vi "Measurement UI.vi"() -> ()   [LabVIEW 2021, in "Load Transient Response with Pin Map UI.lvlib"]
uses:
  Load Transient Response with Pin Map UI.lvlib
  common/builds/PMIC Common.lvlibp/UI/controls/Open Dialog.ctl
  <instrlib>/niScope/Controls/niScope vertical coupling.ctl
  common/builds/PMIC Common.lvlibp/UI/controls/UI Scope Parameters.ctl
  646e44c3-9b14-4556-aaa1-803f5bf26e68.vi
  common/builds/PMIC Common.lvlibp
panel:
  in  "MeasGraphs":T1(tab)
  out "MeasTable":string[][](table)
  out "LoadCurrentV/STimeGraph":waveform(dbl)(graph) caption="Load Transient"
  out "OutputVoltageV/STimeGraph":waveform(dbl)(graph) caption="Load Transient"
  in  "Load Current v/s Time":string="LOAD CURRENT vs TIME"
  in  "Output Voltage v/s Time":string="LOAD VOLTAGE vs TIME"
  out "ScopeGraph":T2(graph)
  out "waveform pins":string[](array[string])
  in  "enforce realtime":bool[](array[boolean])
  in  "reference position":dbl[](array[numeric]) caption="MIN SAMPLE RATE"
  in  "channel enabled":bool[](array[boolean])
  out "waveform length array":i32[](array[numeric])
  out "waveform dt array":dbl[](array[numeric])
  out "concatenated waveform Y":dbl[](array[numeric])
  out "waveform t0 array":dbl[](array[numeric])
  out "waveform sites":i32[](array[numeric])
  in  "vertical range":dbl[](array[numeric]) caption="VERTICAL RANGE"
  in  "vertical offset":dbl[](array[numeric]) caption="VERTICAL OFFSET"
  in  "probe attenuation":dbl[](array[numeric]) caption="PROBE ATTENUATION"
  in  "vertical coupling":T3[](array[typedef]) caption="VERTICAL COUPLING" items=["AC", "DC", "Ground"]
  in  "input impedance":u32[](array[ring]) caption="INPUT IMPEDANCE" items=["1 mega ohm"=0, "50 ohms"=2]
  in  "max input frequency":dbl[](array[numeric]) caption="MAX INPUT FREQUENCY"
  in  "min sample rate":dbl[](array[numeric]) caption="MIN SAMPLE RATE"
  in  "min record length":i32[](array[numeric]) caption="MIN RECORD LENGTH"
  in  "Pin Names for Scope":string[](array[string]) caption="PIN NAMES"
  out "Overshoot load voltage":dbl
  out "Undershoot load voltage":dbl
  out "dt":dbl
  out "Load voltages":dbl[](array[numeric])
  out "Load currents":dbl[](array[numeric])
  in  "Source transient response":i32(ring)=1042 items=["Slow"=1041, "Normal"=1038, "Fast"=1039, "Custom"=1042]
  in  "Load transient response":i32(ring)=3 items=["Slow"=1041, "Normal"=1038, "Fast"=1039, "Custom"=1042]
  in  "Open Dialog":T4
  in  "Scope configuration":string="Scope configuration"
  in  "Load pin name":string caption="LOAD PIN NAME"
  in  "Source pin name":string caption="SOURCE PIN NAME"
  in  "Load sense":i32(ring)=1009 caption="SENSE" items=["Local"=1008, "Remote"=1009]
  in  "Source sense":i32(ring)=1009 caption="SENSE" items=["Local"=1008, "Remote"=1009]
  in  "Load current delay t2":dbl=0.001 caption="DELAY T2" format="%#_6ps"
  in  "Load current delay t1":dbl=0.001 caption="DELAY T1" format="%#_6ps"
  in  "Load current pulse duration":dbl=0.001 caption="PULSE DURATION" format="%#_6ps"
  in  "Load current level range":dbl=40.0 caption="CURRENT LEVEL RANGE" format="%#_6pA"
  in  "Load current rising slew rate":dbl=24.0 caption="CURRENT RISING SLEW RATE" format="%#_6pA/us"
  in  "Load current falling slew rate":dbl=24.0 caption="CURRENT FALLING SLEW RATE" format="%#_6pA/us"
  in  "Load configuration":string="Load configuration"
  in  "Source configuration":string="Source configuration"
  in  "Source voltage level":dbl=12.0 caption="VOLTAGE LEVEL" format="%#_6pV"
  in  "Source current limit":dbl=25.0 caption="CURRENT LIMIT" format="%#_6pA"
  in  "Source voltage pole-zero ratio":dbl=2.0 caption="POLE-ZERO RATIO"
  in  "Source voltage gain bandwidth":dbl=2000.0 caption="GAIN BANDWIDTH" format="%#_6pHz"
  in  "Source voltage compensation frequency":dbl=3530.0 caption="COMP. FREQUENCY" format="%#_6pHz"
  in  "Source fast":bool
  in  "Source normal":bool
  in  "Source slow":bool
  in  "Source SourceAdapt":string="Voltage SourceAdapt Parameters"
  in  "Load voltage limit range":dbl=6.0 caption="VOLTAGE LIMIT RANGE" format="%#_6pV"
  in  "Load current set point 1":dbl=4.0 caption="CURRENT SET POINT 1" format="%#_6pA"
  in  "Load current pole-zero ratio":dbl=0.3 caption="POLE-ZERO RATIO"
  in  "Load current gain bandwidth":dbl=14000.0 caption="GAIN BANDWIDTH" format="%#_6pHz"
  in  "Load current compensation frequency":dbl=180000.0 caption="COMP. FREQUENCY" format="%#_6pHz"
  in  "Load sample rate":dbl=1800000.0 caption="SAMPLE RATE" format="%#_6pS/s"
  in  "Load current set point 2":dbl=14.0 caption="CURRENT SET POINT 2" format="%#_6pA"
  in  "Load fast":bool
  in  "Load normal":bool
  in  "Load slow":bool
  in  "Load SourceAdapt":string="Current SourceAdapt Parameters"
  out "Status":string
  in  "DUT setup time":dbl=1.0 caption="DUT SETUP TIME" format="%#_6ps"
  in  "Measurement settings":string="Measurement settings"
  in  "Nominal output voltage":dbl=3.3 caption="NOMINAL OUTPUT VOLTAGE" format="%#_6pV"
  in  "Mode of operation":T5(ring)=enum."Perform measurement" caption="MODE OF OPERATION"
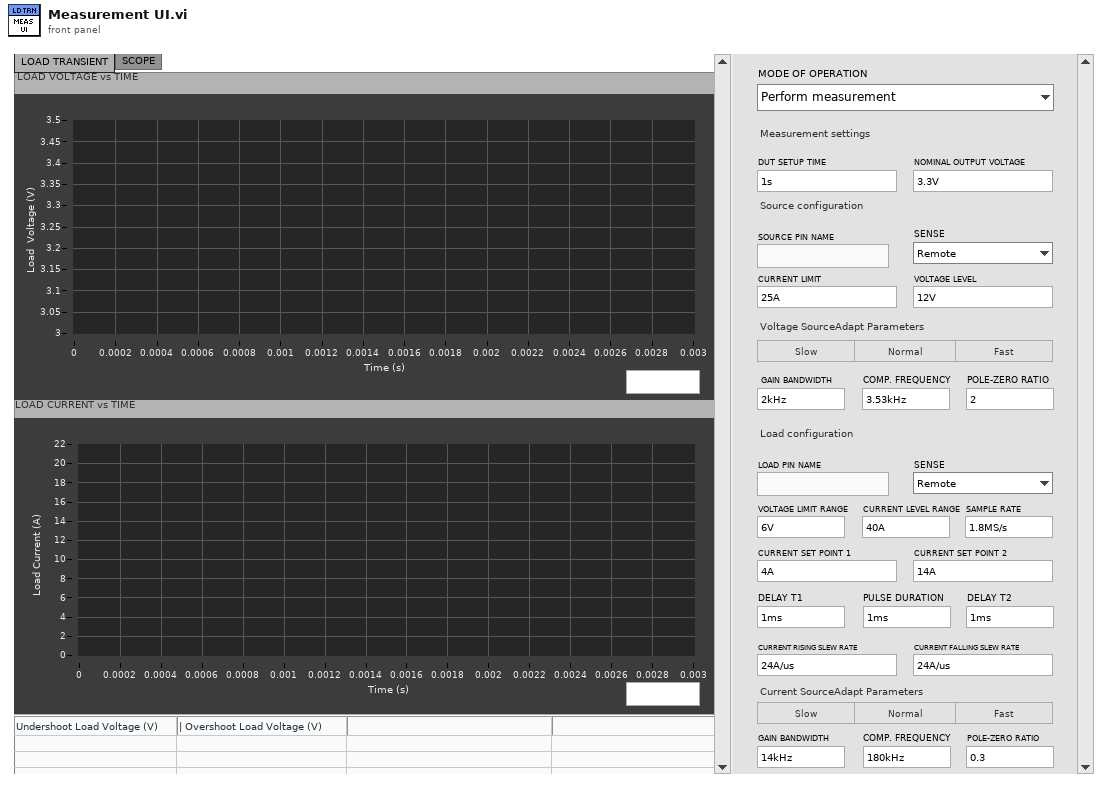
[diagram p1: front panel]
types:
  T1 = enum32{"LOAD TRANSIENT", "SCOPE", "Hidden Controls"}
  T2 = cluster{"Load currents":dbl[], "Efficiency":dbl[]}[]
  T3 = typedef "niScope vertical coupling.ctl" = i32
  T4 = typedef "PMIC Common.lvlibp/Open Dialog.ctl" = bool
  T5 = enum32{"Power on the DUT", "Perform measurement", "Power off the DUT"}
  T6 = typedef "PMIC Common.lvlibp/UI Scope Parameters.ctl" = cluster{"Pin name":string, "Vertical range":dbl, "Vertical offset":dbl, "Probe attenuation":dbl, "Vertical coupling":i32, "Channel enabled":bool, "Input impedance":u32, "Max input frequency":dbl, "Min sample rate":dbl, "Reference position":dbl, "Min record length":i32, "Enforce realtime":bool}
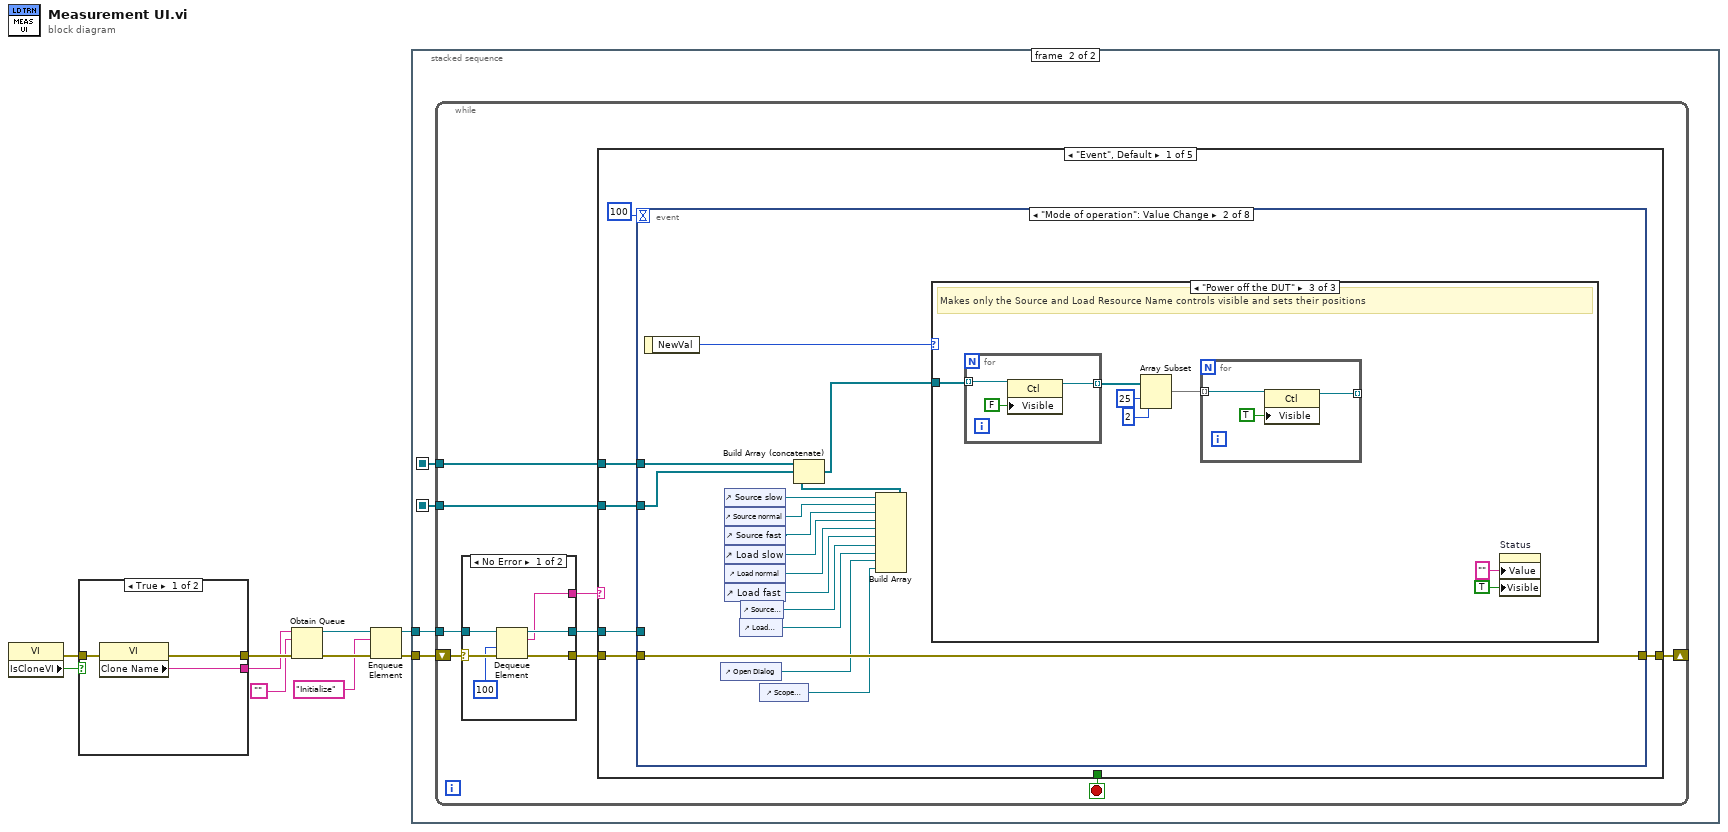
[diagram p0: block diagram]
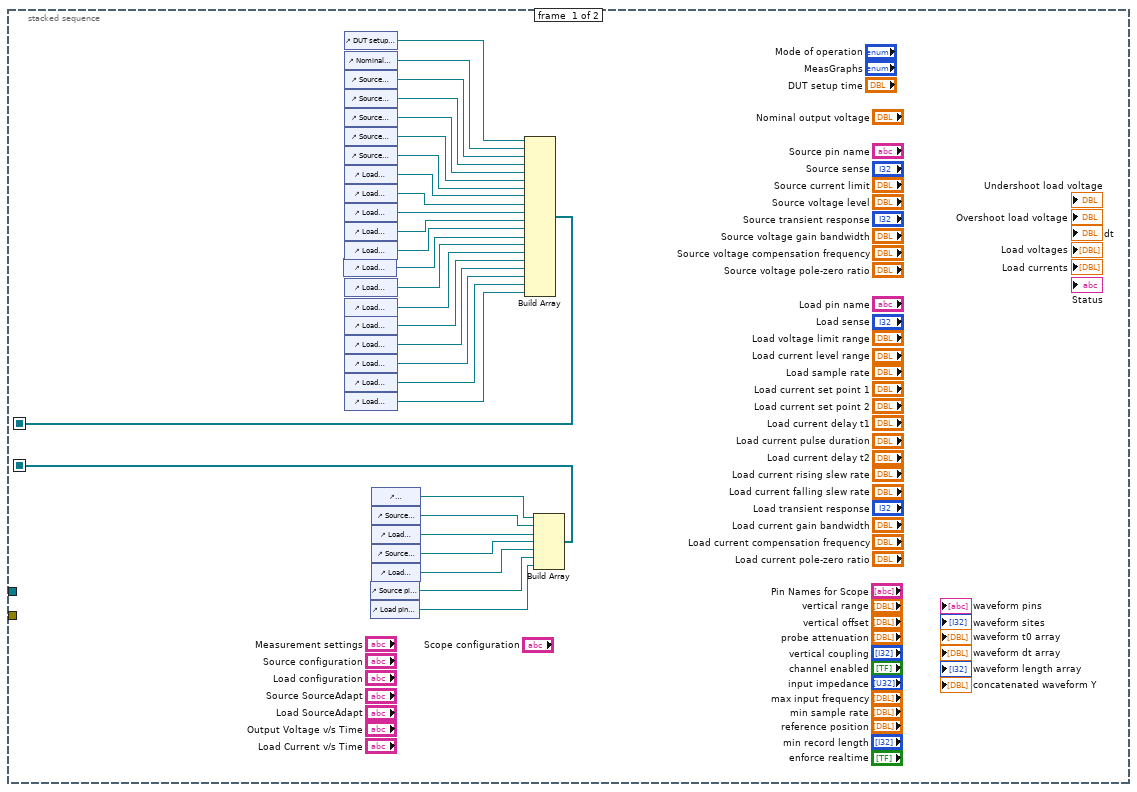
[diagram p2: hidden frame]
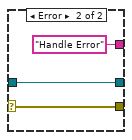
[diagram p3: hidden frame]
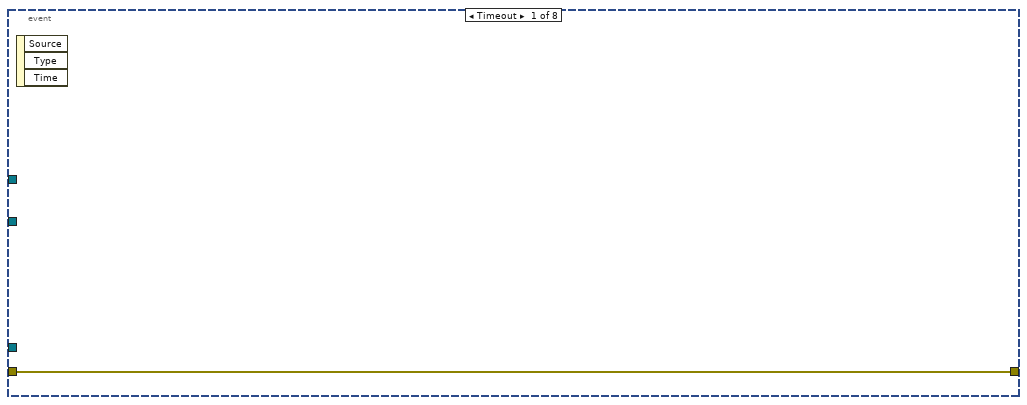
[diagram p4: hidden frame]
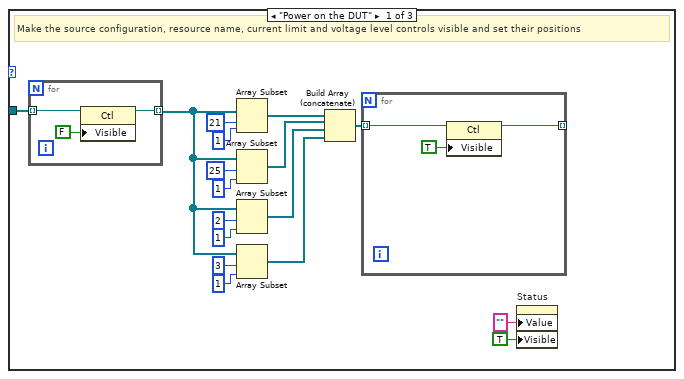
[diagram p5: hidden frame]
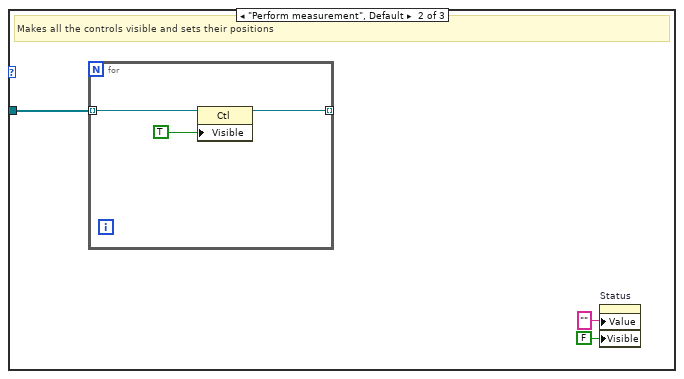
[diagram p6: hidden frame]
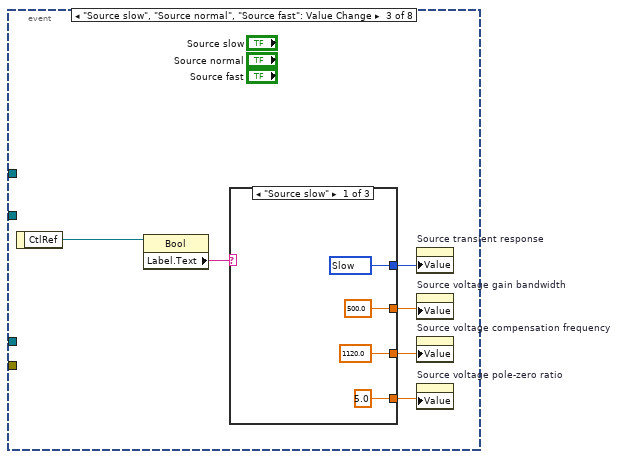
[diagram p7: hidden frame]
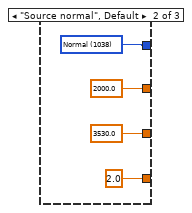
[diagram p8: hidden frame]
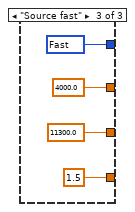
[diagram p9: hidden frame]
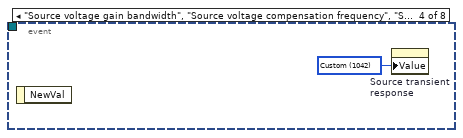
[diagram p10: hidden frame]
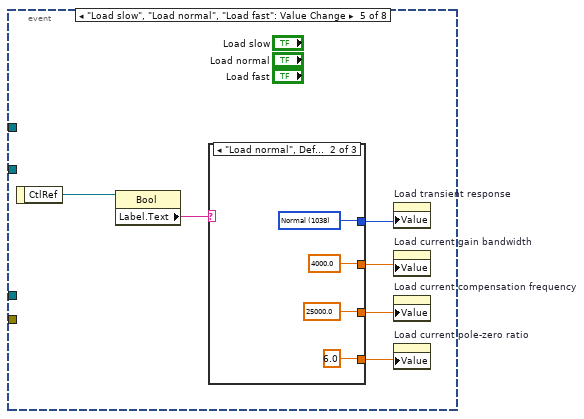
[diagram p11: hidden frame]
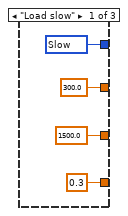
[diagram p12: hidden frame]
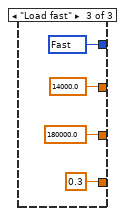
[diagram p13: hidden frame]
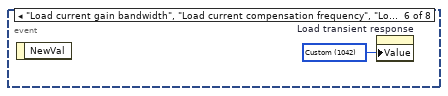
[diagram p14: hidden frame]
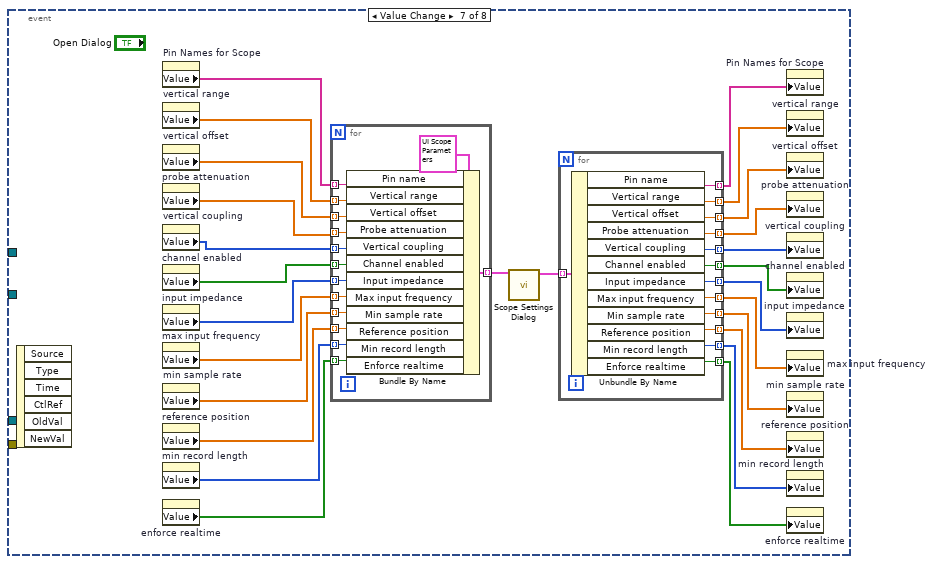
[diagram p15: hidden frame]
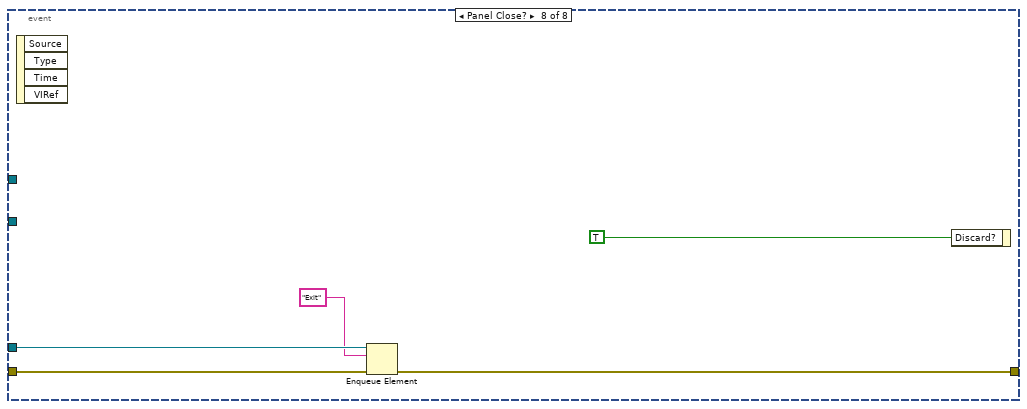
[diagram p16: hidden frame]
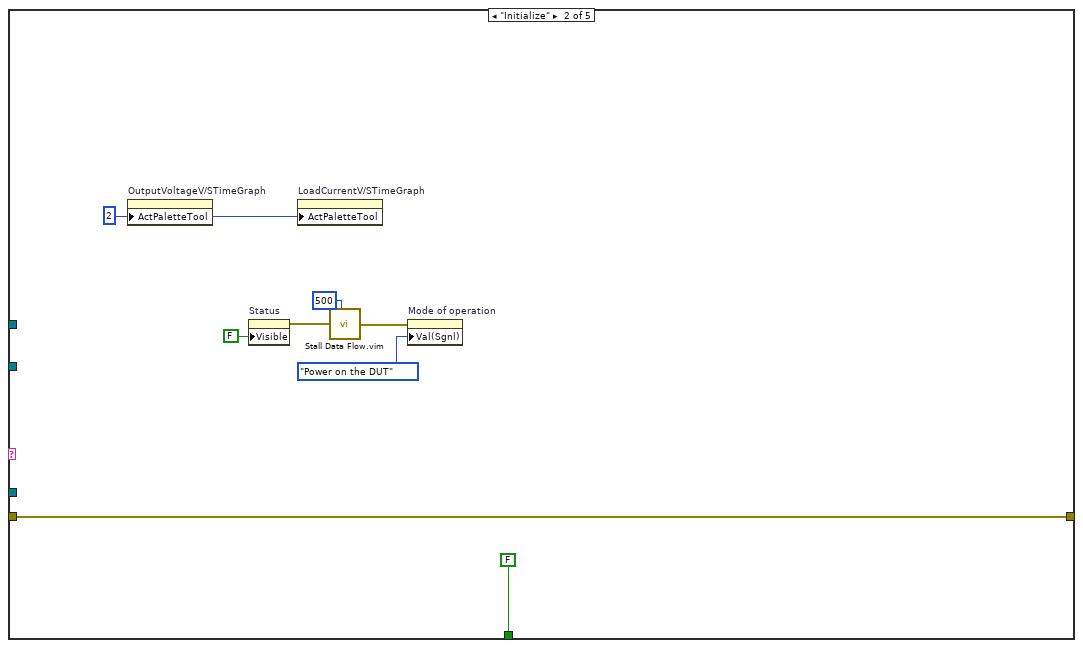
[diagram p17: hidden frame]
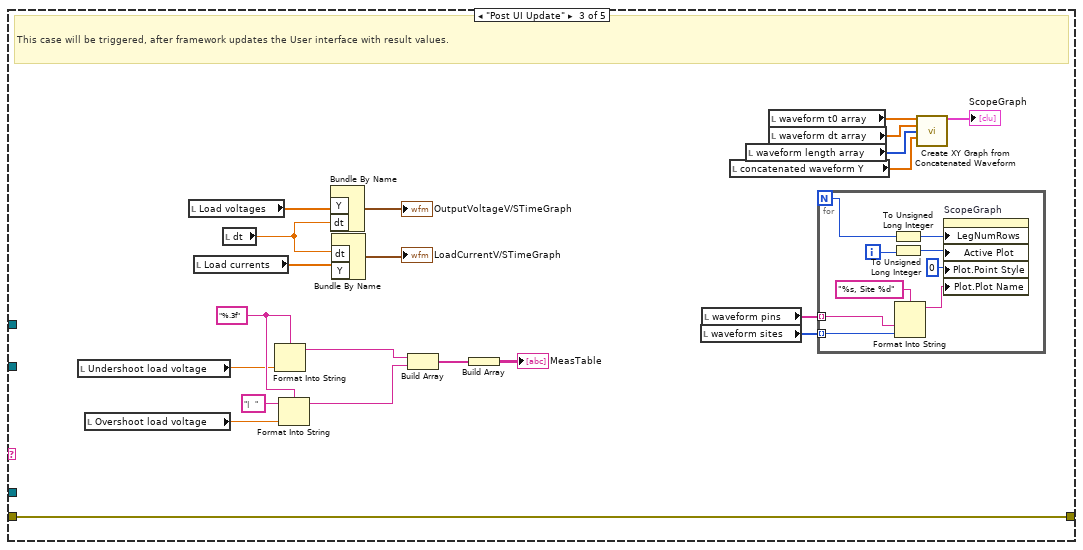
[diagram p18: hidden frame]
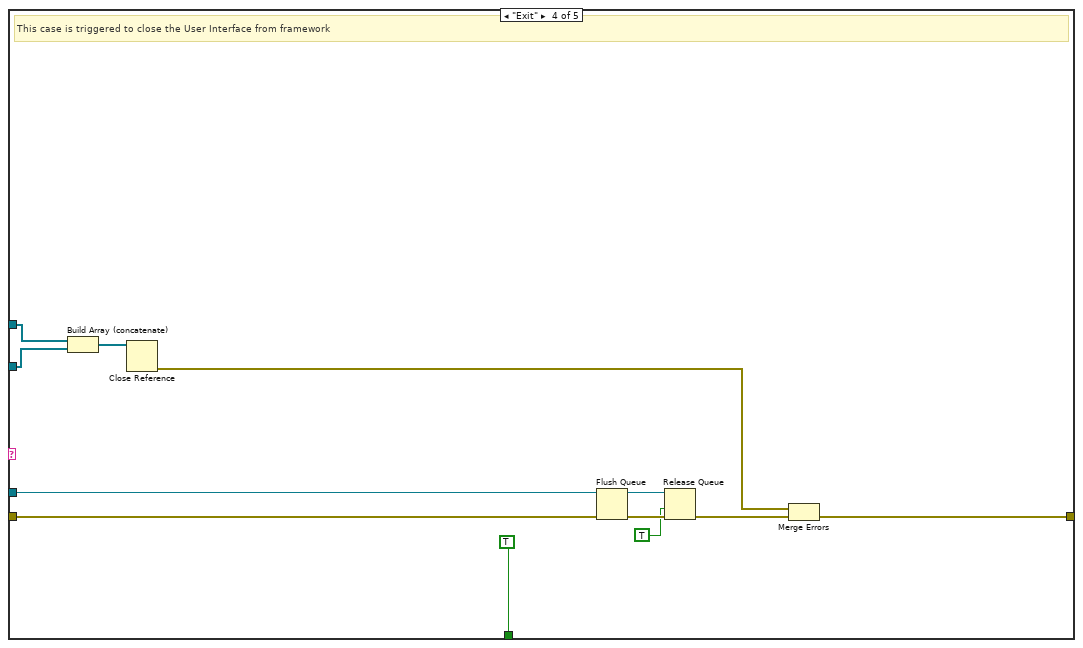
[diagram p19: hidden frame]
diagram:
  n1 = property class="VI"() -> (error out=w1:errorcluster, "IsCloneVI"=w2:bool)  [unwired: 2 in, 1 out]
  n2 = case shown="True" w2 {
    tunnel: [w13 w16] -> w10
    tunnel: [w12 w15] -> w9
    tunnel: w1 -> [w11 w14]
    frame True {
      n3 = property class="VI"(error in=w11) -> (error out=w13:errorcluster, "Clone Name"=w12:string)  [unwired: 1 in, 1 out]
    }
    frame False {
      n4 = property class="VI"(error in=w14) -> (error out=w16:errorcluster, "Name"=w15:string)  [unwired: 1 in, 1 out]
    }
  }
  n5 = Obtain Queue(name (unnamed)=w9, element data type="", error in (no error)=w10) -> (queue out=w6:refnum<queue>, error out=w8:errorcluster)  [unwired: 2 in, 1 out]
  n6 = Enqueue Element(queue=w6, element="Initialize", error in (no error)=w8) -> (queue out=w5:refnum<queue>, error out=w7:errorcluster)  [unwired: 1 in, 1 out]
  n7 = stacked-sequence {
    seq-local: [w31 _] -> [_ w47]
    seq-local: [w32 _] -> [_ w46]
    tunnel: w7 -> [_ w49]
    tunnel: w5 -> [_ w48]
    frame #0 {
      n8 = control-ref of="Load current delay t1"() -> (w21:refnum<vi>)
      n9 = control-ref of="DUT setup time"() -> (w24:refnum<vi>)
      n10 = control-ref of="Nominal output voltage"() -> (w45:refnum<vi>)
      n11 = control-ref of="Source current limit"() -> (w44:refnum<vi>)
      n12 = control-ref of="Source voltage level"() -> (w43:refnum<vi>)
      n13 = control-ref of="Source voltage gain bandwidth"() -> (w42:refnum<vi>)
      n14 = control-ref of="Source voltage compensation frequency"() -> (w41:refnum<vi>)
      n15 = control-ref of="Source voltage pole-zero ratio"() -> (w40:refnum<vi>)
      n16 = control-ref of="Load voltage limit range"() -> (w39:refnum<vi>)
      n17 = control-ref of="Load current level range"() -> (w26:refnum<vi>)
      n18 = control-ref of="Load sample rate"() -> (w38:refnum<vi>)
      n19 = control-ref of="Load current set point 1"() -> (w37:refnum<vi>)
      n20 = control-ref of="Load current set point 2"() -> (w36:refnum<vi>)
      n21 = control-ref of="Load current pulse duration"() -> (w20:refnum<vi>)
      n22 = control-ref of="Load current delay t2"() -> (w19:refnum<vi>)
      n23 = control-ref of="Load current rising slew rate"() -> (w22:refnum<vi>)
      n24 = control-ref of="Load current falling slew rate"() -> (w23:refnum<vi>)
      n25 = control-ref of="Load current gain bandwidth"() -> (w25:refnum<vi>)
      n26 = control-ref of="Load current compensation frequency"() -> (w35:refnum<vi>)
      n27 = control-ref of="Load current pole-zero ratio"() -> (w33:refnum<vi>)
      n28 = control-ref of="Source pin name"() -> (w18:refnum<vi>)
      n29 = control-ref of="Load pin name"() -> (w17:refnum<vi>)
      n30 = control-ref of="Measurement settings"() -> (w34:refnum<vi>)
      n31 = control-ref of="Source configuration"() -> (w30:refnum<vi>)
      n32 = control-ref of="Load configuration"() -> (w29:refnum<vi>)
      n33 = control-ref of="Source SourceAdapt"() -> (w28:refnum<vi>)
      n34 = control-ref of="Load SourceAdapt"() -> (w27:refnum<vi>)
      n35 = Build Array(w24, w45, w44, w43, w42, w41, w40, w39, w26, w38, w37, w36, w21, w20, w19, w22, w23, w25, w35, w33) -> (w31:refnum<vi>[])
      n36 = Build Array(w34, w30, w29, w28, w27, w18, w17) -> (w32:refnum<vi>[])
    }
    frame #1 {
      n37 = while {
        shift-right: [w53] -> _
        shift-left: w49 -> [w58]
        tunnel: w48 -> [w56]
        tunnel: w47 -> [w51]
        tunnel: w46 -> [w50]
        stop <- w52 stop-if-true
        n38 = case shown="No Error" w58 {
          selector: w58 -> [w64 w67]
          tunnel: [w63 w67] -> w57
          tunnel: w56 -> [w62 w66]
          tunnel: [w61 w66] -> w55
          tunnel: [w60 "Handle Error"] -> w54
          frame No Error {
            n39 = Dequeue Element(queue=w62, timeout in ms (-1)=100, error in (no error)=w64) -> (queue out=w61:refnum<queue>, element=w60:string, error out=w63:errorcluster)  [unwired: 1 out]
          }
          frame Error {
          }
        }
        n40 = case shown="\"Event\", Default" w54 {
          tunnel: w57 -> [w72 w236 w257 w278 w279]
          tunnel: w55 -> [w70 _ _ w276 _]
          tunnel: [w73 w236 w257 w267 w279] -> w53
          tunnel: [_ FALSE _ TRUE _] -> w52
          tunnel: w51 -> [w69 _ _ w272 _]
          tunnel: w50 -> [w68 _ _ w271 _]
          frame "Event", Default {
            n41 = event shown="[1] \"Mode of operation\": Value Change" {
              selector: _ -> [_ _ _ _ _ _ _ _]
              dyn-events: _ -> [_ _ _ _ _ _ _ _]
              timeout: 100 -> [_ _ _ _ _ _ _ _]
              tunnel: [w74 w86 _ _ _ _ _ w226] -> w73
              tunnel: w72 -> [w74 w86 _ _ _ _ _ w227]
              tunnel: w70 -> [_ _ _ _ _ _ _ w225]
              tunnel: w69 -> [_ w88 _ _ _ _ _ _]
              tunnel: w68 -> [_ w87 _ _ _ _ _ _]
              event Timeout {
                n42 = event-data() -> ()  [unwired: 1 in, 3 out]
              }
              event "Mode of operation": Value Change {
                n43 = event-data() -> ("NewVal"=w90:T5)  [unwired: 1 in]
                n44 = control-ref of="Open Dialog"() -> (w76:refnum<vi>)
                n45 = control-ref of="Source slow"() -> (w85:refnum<vi>)
                n46 = control-ref of="Source normal"() -> (w84:refnum<vi>)
                n47 = control-ref of="Source fast"() -> (w80:refnum<vi>)
                n48 = control-ref of="Load slow"() -> (w83:refnum<vi>)
                n49 = control-ref of="Load normal"() -> (w82:refnum<vi>)
                n50 = control-ref of="Load fast"() -> (w81:refnum<vi>)
                n51 = control-ref of="Load sense"() -> (w77:refnum<vi>)
                n52 = control-ref of="Source sense"() -> (w78:refnum<vi>)
                n53 = control-ref of="Scope configuration"() -> (w75:refnum<vi>)
                n54 = Build Array(w85, w84, w80, w83, w82, w81, w78, w77, w76, w75) -> (w79:refnum<vi>[])
                n55 = Build Array (concatenate)(w88, w87, w79) -> (w89:refnum<vi>[])
                n56 = case shown="\"Power off the DUT\"" w90 {
                  tunnel: w89 -> [w93 w116 w124]
                  frame "Power on the DUT" {
                    # "Make the source configuration, resource name, current limit and voltage level controls visible and set their positions"
                    n57 = for {
                      tunnel: w93 -> [w110] mode=indexing
                      tunnel: [w108] -> w104 mode=indexing
                      n58 = property class="Ctl"(reference=w110, "Visible"=FALSE) -> (reference out=w108:refnum<vi>)  [unwired: 1 in, 1 out]
                    }
                    n59 = Array Subset(array=w104, index=21 ("length"), length=1 ("index")) -> (w102:refnum<vi>[])
                    n60 = Array Subset(array=w104, index=25 ("length"), length=1 ("index")) -> (w103:refnum<vi>[])
                    n61 = Array Subset(array=w104, index=2 ("length"), length=1 ("index")) -> (w105:refnum<vi>[])
                    n62 = Array Subset(array=w104, index=3 ("length"), length=1 ("index")) -> (w107:refnum<vi>[])
                    n63 = Build Array (concatenate)(w102, w103, w105, w107) -> (w106:refnum<vi>[])
                    n64 = for {
                      tunnel: [w112] -> _ mode=indexing
                      tunnel: w106 -> [w111] mode=indexing
                      n65 = property class="Ctl"(reference=w111, "Visible"=TRUE) -> (reference out=w112:refnum<vi>)  [unwired: 1 in, 1 out]
                    }
                    n66 = property on="Status" class="Str"("Value"="" ("Status"), "Visible"=TRUE) -> ()  [unwired: 2 in, 2 out]
                  }
                  frame "Perform measurement", Default {
                    # "Makes all the controls visible and sets their positions"
                    n67 = for {
                      tunnel: w116 -> [w117] mode=indexing
                      tunnel: [w118] -> _ mode=indexing
                      n68 = property class="Ctl"(reference=w117, "Visible"=TRUE) -> (reference out=w118:refnum<vi>)  [unwired: 1 in, 1 out]
                    }
                    n69 = property on="Status" class="Str"("Value"="" ("Operation"), "Visible"=FALSE) -> ()  [unwired: 2 in, 2 out]
                  }
                  frame "Power off the DUT" {
                    # "Makes only the Source and Load Resource Name controls visible and sets their positions"
                    n70 = for {
                      tunnel: w124 -> [w128] mode=indexing
                      tunnel: [w127] -> w121 mode=indexing
                      n71 = property class="Ctl"(reference=w128, "Visible"=FALSE) -> (reference out=w127:refnum<vi>)  [unwired: 1 in, 1 out]
                    }
                    n72 = Array Subset(array=w121, index=25 ("length"), length=2 ("index")) -> (w120:refnum<vi>[])
                    n73 = for {
                      tunnel: w120 -> [w130] mode=indexing
                      tunnel: [w131] -> _ mode=indexing
                      n74 = property class="Ctl"(reference=w130, "Visible"=TRUE) -> (reference out=w131:refnum<vi>)  [unwired: 1 in, 1 out]
                    }
                    n75 = property on="Status" class="Str"("Value"="" ("Status"), "Visible"=TRUE) -> ()  [unwired: 2 in, 2 out]
                  }
                }
              }
              event "Source slow", "Source normal", "Source fast": Value Change {
                n76 = event-data() -> ("CtlRef"=w138:refnum<vi>)  [unwired: 1 in]
                n77 = property class="Bool"(reference=w138) -> ("Label.Text"=w137:string)  [unwired: 1 in, 2 out]
                n78 = case shown="\"Source slow\"" w137 {
                  tunnel: [w142 w146 w150] -> w136
                  tunnel: [500.0 ("Source voltage gain bandwidth") 2000.0 ("Source voltage gain bandwidth") 4000.0 ("Source voltage gain bandwidth")] -> w135
                  tunnel: [1120.0 ("Source voltage compensation frequency") 3530.0 ("Source voltage compensation frequency") 11300.0 ("Source voltage compensation frequency")] -> w134
                  tunnel: [5.0 ("Source voltage pole-zero ratio") 2.0 ("Source voltage pole-zero ratio") 1.5 ("Source voltage pole-zero ratio")] -> w133
                  frame "Source slow" {
                    w142 = 1041 items=["Slow"=1041, "Normal"=1038, "Fast"=1039, "Custom"=1042] ("Source transient response")
                  }
                  frame "Source normal", Default {
                    w146 = 1038 items=["Slow"=1041, "Normal"=1038, "Fast"=1039, "Custom"=1042] ("Source transient response")
                  }
                  frame "Source fast" {
                    w150 = 1039 items=["Slow"=1041, "Normal"=1038, "Fast"=1039, "Custom"=1042] ("Source transient response")
                  }
                }
                n79 = property on="Source transient response" class="Ring (strict)"("Value"=w136) -> ()  [unwired: 2 in, 2 out]
                n80 = property on="Source voltage gain bandwidth" class="DigNum (strict)"("Value"=w135) -> ()  [unwired: 2 in, 2 out]
                n81 = property on="Source voltage compensation frequency" class="DigNum (strict)"("Value"=w134) -> ()  [unwired: 2 in, 2 out]
                n82 = property on="Source voltage pole-zero ratio" class="DigNum (strict)"("Value"=w133) -> ()  [unwired: 2 in, 2 out]
              }
              event "Source voltage gain bandwidth", "Source voltage compensation frequency", "Source voltage pole-zero ratio": Value Change {
                w151 = 1042 items=["Slow"=1041, "Normal"=1038, "Fast"=1039, "Custom"=1042] ("Source transient response")
                n83 = event-data() -> ()  [unwired: 1 in, 1 out]
                n84 = property on="Source transient response" class="Ring (strict)"("Value"=w151) -> ()  [unwired: 2 in, 2 out]
              }
              event "Load slow", "Load normal", "Load fast": Value Change {
                n85 = event-data() -> ("CtlRef"=w156:refnum<vi>)  [unwired: 1 in]
                n86 = property class="Bool"(reference=w156) -> ("Label.Text"=w157:string)  [unwired: 1 in, 2 out]
                n87 = case shown="\"Load normal\", Default" w157 {
                  tunnel: [w161 w165 w169] -> w155
                  tunnel: [300.0 ("Load current gain bandwidth") 4000.0 ("Load current gain bandwidth") 14000.0 ("Load current gain bandwidth")] -> w154
                  tunnel: [1500.0 ("Load current compensation frequency") 25000.0 ("Load current compensation frequency") 180000.0 ("Load current compensation frequency")] -> w153
                  tunnel: [0.3 ("Load current pole-zero ratio") 6.0 ("Load current pole-zero ratio") 0.3 ("Load current pole-zero ratio")] -> w152
                  frame "Load slow" {
                    w161 = 1041 items=["Slow"=1041, "Normal"=1038, "Fast"=1039, "Custom"=1042] ("Source transient response")
                  }
                  frame "Load normal", Default {
                    w165 = 1038 items=["Slow"=1041, "Normal"=1038, "Fast"=1039, "Custom"=1042] ("Source transient response")
                  }
                  frame "Load fast" {
                    w169 = 1039 items=["Slow"=1041, "Normal"=1038, "Fast"=1039, "Custom"=1042] ("Source transient response")
                  }
                }
                n88 = property on="Load transient response" class="Ring (strict)"("Value"=w155) -> ()  [unwired: 2 in, 2 out]
                n89 = property on="Load current gain bandwidth" class="DigNum (strict)"("Value"=w154) -> ()  [unwired: 2 in, 2 out]
                n90 = property on="Load current compensation frequency" class="DigNum (strict)"("Value"=w153) -> ()  [unwired: 2 in, 2 out]
                n91 = property on="Load current pole-zero ratio" class="DigNum (strict)"("Value"=w152) -> ()  [unwired: 2 in, 2 out]
              }
              event "Load current gain bandwidth", "Load current compensation frequency", "Load current pole-zero ratio": Value Change {
                w170 = 1042 items=["Slow"=1041, "Normal"=1038, "Fast"=1039, "Custom"=1042] ("Load transient response")
                n92 = event-data() -> ()  [unwired: 1 in, 1 out]
                n93 = property on="Load transient response" class="Ring (strict)"("Value"=w170) -> ()  [unwired: 2 in, 2 out]
              }
              event Value Change {
                n94 = event-data() -> ()  [unwired: 1 in, 6 out]
                n95 = property on="Pin Names for Scope" class="Arr (strict)"() -> ("Value"=w195:string[])  [unwired: 2 in, 2 out]
                n96 = property on="vertical range" class="Arr (strict)"() -> ("Value"=w194:dbl[])  [unwired: 2 in, 2 out]
                n97 = property on="vertical offset" class="Arr (strict)"() -> ("Value"=w193:dbl[])  [unwired: 2 in, 2 out]
                n98 = property on="probe attenuation" class="Arr (strict)"() -> ("Value"=w192:dbl[])  [unwired: 2 in, 2 out]
                n99 = property on="vertical coupling" class="Arr (strict)"() -> ("Value"=w191:T3[])  [unwired: 2 in, 2 out]
                n100 = property on="channel enabled" class="Arr (strict)"() -> ("Value"=w190:bool[])  [unwired: 2 in, 2 out]
                n101 = property on="input impedance" class="Arr (strict)"() -> ("Value"=w189:u32[])  [unwired: 2 in, 2 out]
                n102 = property on="max input frequency" class="Arr (strict)"() -> ("Value"=w188:dbl[])  [unwired: 2 in, 2 out]
                n103 = property on="min sample rate" class="Arr (strict)"() -> ("Value"=w187:dbl[])  [unwired: 2 in, 2 out]
                n104 = property on="reference position" class="Arr (strict)"() -> ("Value"=w186:dbl[])  [unwired: 2 in, 2 out]
                n105 = property on="min record length" class="Arr (strict)"() -> ("Value"=w185:i32[])  [unwired: 2 in, 2 out]
                n106 = property on="enforce realtime" class="Arr (strict)"() -> ("Value"=w184:bool[])  [unwired: 2 in, 2 out]
                n107 = for {
                  tunnel: [w222] -> w196 mode=indexing
                  tunnel: w195 -> [w221] mode=indexing
                  tunnel: w194 -> [w220] mode=indexing
                  tunnel: w193 -> [w219] mode=indexing
                  tunnel: w192 -> [w218] mode=indexing
                  tunnel: w191 -> [w217] mode=indexing
                  tunnel: w190 -> [w216] mode=indexing
                  tunnel: w189 -> [w215] mode=indexing
                  tunnel: w188 -> [w214] mode=indexing
                  tunnel: w187 -> [w213] mode=indexing
                  tunnel: w186 -> [w212] mode=indexing
                  tunnel: w185 -> [w211] mode=indexing
                  tunnel: w184 -> [w210] mode=indexing
                  n108 = Bundle By Name(cluster=T6 {"Pin name"="", "Vertical range"=10.0, "Vertical offset"=0.0, "Probe attenuation"=1.0, "Vertical coupling"=1, "Channel enabled"=TRUE, "Input impedance"=0, "Max input frequency"=0.0, "Min sample rate"=20000000.0, "Reference position"=50.0, "Min record length"=1000, "Enforce realtime"=TRUE} ("Scope Parameters"), "Pin name"=w221, "Vertical range"=w220, "Vertical offset"=w219, "Probe attenuation"=w218, "Vertical coupling"=w217, "Channel enabled"=w216, "Input impedance"=w215, "Max input frequency"=w214, "Min sample rate"=w213, "Reference position"=w212, "Min record length"=w211, "Enforce realtime"=w210) -> (w222:T6)
                }
                n109 = call "Scope Settings Dialog.vi"("Scope Parameters"=w196) -> ("Scope Parameters out"=w183:T6[])  [unwired: 10 in]
                n110 = for {
                  tunnel: w183 -> [w209] mode=indexing
                  tunnel: [w208] -> w182 mode=indexing
                  tunnel: [w207] -> w181 mode=indexing
                  tunnel: [w206] -> w180 mode=indexing
                  tunnel: [w205] -> w179 mode=indexing
                  tunnel: [w204] -> w178 mode=indexing
                  tunnel: [w203] -> w177 mode=indexing
                  tunnel: [w202] -> w176 mode=indexing
                  tunnel: [w201] -> w175 mode=indexing
                  tunnel: [w200] -> w174 mode=indexing
                  tunnel: [w199] -> w173 mode=indexing
                  tunnel: [w198] -> w172 mode=indexing
                  tunnel: [w197] -> w171 mode=indexing
                  n111 = Unbundle By Name(w209) -> ("Pin name"=w208:string, "Vertical range"=w207:dbl, "Vertical offset"=w206:dbl, "Probe attenuation"=w205:dbl, "Vertical coupling"=w204:i32, "Channel enabled"=w203:bool, "Input impedance"=w202:u32, "Max input frequency"=w201:dbl, "Min sample rate"=w200:dbl, "Reference position"=w199:dbl, "Min record length"=w198:i32, "Enforce realtime"=w197:bool)
                }
                n112 = property on="Pin Names for Scope" class="Arr (strict)"("Value"=w182) -> ()  [unwired: 2 in, 2 out]
                n113 = property on="vertical range" class="Arr (strict)"("Value"=w181) -> ()  [unwired: 2 in, 2 out]
                n114 = property on="vertical offset" class="Arr (strict)"("Value"=w180) -> ()  [unwired: 2 in, 2 out]
                n115 = property on="probe attenuation" class="Arr (strict)"("Value"=w179) -> ()  [unwired: 2 in, 2 out]
                n116 = property on="vertical coupling" class="Arr (strict)"("Value"=w178) -> ()  [unwired: 2 in, 2 out]
                n117 = property on="channel enabled" class="Arr (strict)"("Value"=w177) -> ()  [unwired: 2 in, 2 out]
                n118 = property on="input impedance" class="Arr (strict)"("Value"=w176) -> ()  [unwired: 2 in, 2 out]
                n119 = property on="max input frequency" class="Arr (strict)"("Value"=w175) -> ()  [unwired: 2 in, 2 out]
                n120 = property on="min sample rate" class="Arr (strict)"("Value"=w174) -> ()  [unwired: 2 in, 2 out]
                n121 = property on="reference position" class="Arr (strict)"("Value"=w173) -> ()  [unwired: 2 in, 2 out]
                n122 = property on="min record length" class="Arr (strict)"("Value"=w172) -> ()  [unwired: 2 in, 2 out]
                n123 = property on="enforce realtime" class="Arr (strict)"("Value"=w171) -> ()  [unwired: 2 in, 2 out]
              }
              event Panel Close? {
                n124 = event-data() -> ()  [unwired: 1 in, 4 out]
                n125 = Enqueue Element(queue=w225, element="Exit", error in (no error)=w227) -> (error out=w226:errorcluster)  [unwired: 1 in, 2 out]
                n126 = event-data("Discard?"=TRUE) -> ()  [unwired: 1 in, 1 out]
              }
            }
          }
          frame "Initialize" {
            w234 = 2 ("Palette:Active Tool")
            n127 = property on="OutputVoltageV/STimeGraph" class="WFGraph (strict)"("ActPaletteTool"=w234) -> ()  [unwired: 2 in, 2 out]
            n128 = property on="Status" class="Str"("Visible"=FALSE) -> (error out=w231:errorcluster)  [unwired: 2 in, 1 out]
            n129 = property on="LoadCurrentV/STimeGraph" class="WFGraph (strict)"("ActPaletteTool"=w234) -> ()  [unwired: 2 in, 2 out]
            n130 = call "Stall Data Flow.vim"("value in"=w231, "milliseconds to wait"=u32 500) -> ("value out"=w230:errorcluster)  [unwired: 1 out]
            n131 = property on="Mode of operation" class="Enum (strict)"(error in=w230, "Val(Sgnl)"=T5."Power on the DUT" ("Value (Signaling)")) -> ()  [unwired: 1 in, 2 out]
          }
          frame "Post UI Update" {
            w248 = "%.3f" ("initial string")
            # "This case will be triggered, after framework updates the User interface with result values."
            n132 = local read "Undershoot load voltage"() -> (w247:dbl)
            n133 = local read "Overshoot load voltage"() -> (w246:dbl)
            n134 = local read "Load voltages"() -> (w254:dbl[])
            n135 = local read "Load currents"() -> (w253:dbl[])
            n136 = local read "dt"() -> (w252:dbl)
            n137 = Format Into String(format string=w248, w247) -> (resulting string=w245:string)  [unwired: 2 in, 1 out]
            n138 = Format Into String(format string=w248, initial string="|   ", w246) -> (resulting string=w244:string)  [unwired: 1 in, 1 out]
            n139 = Bundle By Name("Y"=w254, "dt"=w252) -> (→"OutputVoltageV/STimeGraph":waveform(dbl))  [unwired: 1 in]
            n140 = Bundle By Name("dt"=w252, "Y"=w253) -> (→"LoadCurrentV/STimeGraph":waveform(dbl))  [unwired: 1 in]
            n141 = Build Array(w245, w244) -> (w250:string[])
            n142 = Build Array(w250) -> (→"MeasTable":string[][])
            n143 = local read "waveform sites"() -> (w238:i32[])
            n144 = local read "waveform pins"() -> (w237:string[])
            n145 = local read "concatenated waveform Y"() -> (w239:dbl[])
            n146 = local read "waveform length array"() -> (w240:i32[])
            n147 = local read "waveform t0 array"() -> (w242:dbl[])
            n148 = local read "waveform dt array"() -> (w241:dbl[])
            n149 = for {
              N -> [w261]
              tunnel: w238 -> [w259] mode=indexing
              tunnel: w237 -> [w258] mode=indexing
              i -> [w262]
              n150 = To Unsigned Long Integer(number=w261) -> (unsigned 32bit integer=w260:u32)
              n151 = To Unsigned Long Integer(number=w262) -> (unsigned 32bit integer=w263:u32)
              n152 = Format Into String(format string="%s, Site %d", w258, w259) -> (resulting string=w265:string)  [unwired: 2 in, 1 out]
              n153 = property on="ScopeGraph" class="XYGraph (strict)"("LegNumRows"=w260, "Active Plot"=w263, "Plot.Point Style"=u8 0, "Plot.Plot Name"=w265) -> ()  [unwired: 2 in, 2 out]
            }
            n154 = call "Create XY Graph from Concatenated Waveform.vi"("waveform t0 array"=w242, "waveform dt array"=w241, "waveform length array"=w240, "concatenated waveform Y"=w239) -> ("XY Graph Array"=→"ScopeGraph":cluster{"time":dbl[], "waveform":dbl[]}[])  [unwired: 11 in]
          }
          frame "Exit" {
            # "This case is triggered to close the User Interface from framework"
            n155 = Build Array (concatenate)(w272, w271) -> (w270:refnum<vi>[])
            n156 = Close Reference(reference=w270) -> (error out=w268:errorcluster)  [unwired: 1 in]
            n157 = Flush Queue(queue=w276, error in (no error)=w278) -> (queue out=w275:refnum<queue>, error out=w274:errorcluster)  [unwired: 1 out]
            n158 = Release Queue(queue=w275, force destroy? (F)=TRUE, error in (no error)=w274) -> (error out=w269:errorcluster)  [unwired: 2 out]
            n159 = Merge Errors(w268, w269) -> (w267:errorcluster)
          }
          frame "Handle Error" {
          }
        }
      }
    }
  }
